vi "Relay Switcher FVT2023.vi"(9 "Address":u8=6, 10 "GPIB":u8, 11 "RF Position":u16=1 min=1 max=63 step=1) -> ()   [LabVIEW 2023]
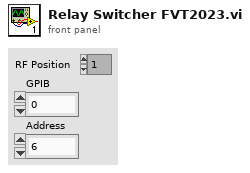
[diagram p1: front panel]
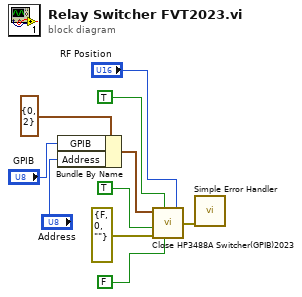
[diagram p0: block diagram]
diagram:
  n1 = Bundle By Name(cluster=cluster{"GPIB":u8, "Address":u8} {"GPIB"=0, "Address"=2} ("Device In"), "GPIB"="GPIB", "Address"="Address") -> (w5:cluster{"GPIB":u8, "Address":u8})
  n2 = call "Close HP3488A Switcher(GPIB)2023.vi"("Device In"=w5, "reset"=TRUE, "Use Card# 5"=TRUE, "ID query"=FALSE, "error in (no error)"=errorcluster {"status"=FALSE, "code"=0, "source"=""}, "Position Number"="RF Position") -> ("error out"=w9:errorcluster)  [unwired: 2 in]
  n3 = call <vilib>:"Simple Error Handler.vi"("error in (no error)"=w9) -> ()  [unwired: 4 in, 5 out]
